vi "RF_SetConnector.vi"(7 "IO Mode":T1 items=["IO", "Output", "Loop", "Input", "Close"], 8 "error in (no error)":errorcluster, 11 "RFIndex":u32) -> (0 "error out":errorcluster, 3 "return":i32)   [LabVIEW 2018]
uses:
  Common/Types/IO Mode.ctl
  Common/Driver/rd.dll
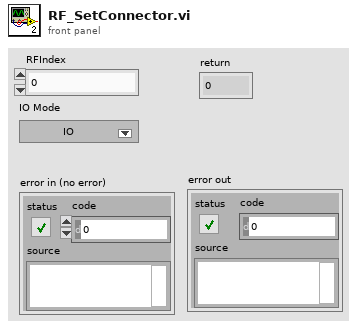
[diagram p1: front panel]
types:
  T1 = typedef "IO Mode.ctl" = u32
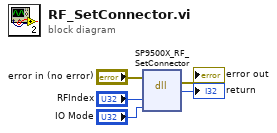
[diagram p0: block diagram]
diagram:
  n1 = dll-call lib="C:/rd/LabVIEW/Common/Driver/rd.dll" fn="SP9500X_RF_SetConnector"(error in="error in (no error)", "RFIndex"="RFIndex", "Connector"="IO Mode") -> (error out=→"error out":errorcluster, "return"=→"return":i32)  [unwired: 4 in, 1 out]
